vi "cDAQ Get Info.vi"(8 "error in":errorcluster, 11 "cdaq session":T1={"mclk [Hz]"=12800000.0, "ADC task"="", "mclk reference"="", "fs [Hz]"=50000.0, "queue adc cmd"=refnum, "queue adc data"=refnum, "adc proc ref"=refnum, "channels"=[], "last channels"=[], "timeout"=timestamp(0 s since 1904-01-01), "N"=1000, "mclk mode"=enum."Free running", "ext mclk source"=""} {"last channels"."Channel id" min=0 step=1; "channels"."Channel id" min=0 step=1}) -> (0 "error out":errorcluster, 2 "needs ext. mclk source?":bool=TRUE)   [LabVIEW 2013]
doc: "Get some infos and flags for given digitizer setup."
uses:
  cDAQ Session.ctl
  low_level_old/cdaq_anal_adc_command.ctl
  low_level_old/cdaq_anal_adc_data.ctl
  cDAQ Virtual Channel.ctl
  cDAQ Master Clock Mode.ctl
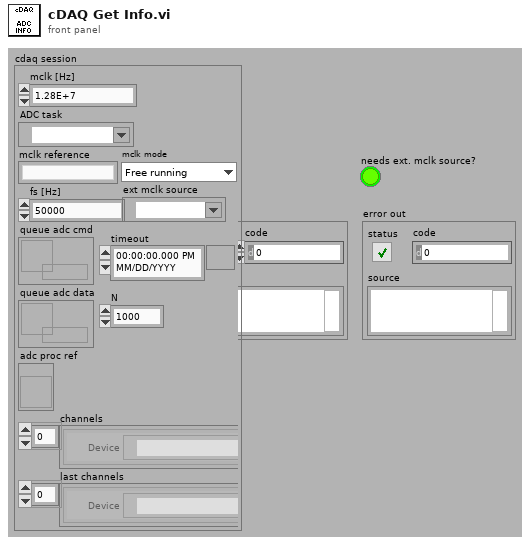
[diagram p1: front panel]
types:
  T1 = typedef "cDAQ Session.ctl" = cluster{"mclk [Hz]":dbl, "ADC task":refnum<k21>, "mclk reference":string, "fs [Hz]":dbl, "queue adc cmd":refnum<queue>, "queue adc data":refnum<queue>, "adc proc ref":refnum<vi>, "channels":T2[], "last channels":T2[], "timeout":timestamp, "N":i32, "mclk mode":T3, "ext mclk source":tag}
  T2 = typedef "cDAQ Virtual Channel.ctl" = cluster{"Device":tag, "Channel id":i32, "btn clr":bool, "btn up":bool, "btn down":bool}
  T3 = typedef "cDAQ Master Clock Mode.ctl" = enum16{"Free running", "Export master clock", "Import master clock"}
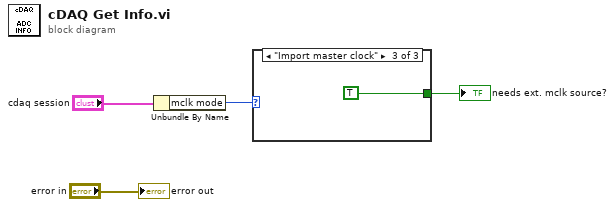
[diagram p0: block diagram]
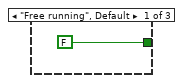
[diagram p2: hidden frame]
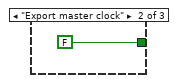
[diagram p3: hidden frame]
diagram:
  n1 = Unbundle By Name("cdaq session") -> ("mclk mode"=w2:T3)
  n2 = case shown="\"Import master clock\"" w2 {
    tunnel: [FALSE FALSE TRUE] -> w1
    frame "Free running", Default {
    }
    frame "Export master clock" {
    }
    frame "Import master clock" {
    }
  }
  "needs ext. mclk source?" <- w1
  "error out" <- "error in"
